vi "TOP画面.vi"() -> ()   [LabVIEW 2021]
uses:
  <vilib>/Utility/config.llb/Read Key (String).vi
  <vilib>/Utility/config.llb/NI_LVConfig.lvlib
panel:
  out "iniフォルダパス取得 2":path
  out "ini error in (no error) 2":errorcluster caption="エラー入力（エラーなし）"
  out "品番設定_品番品名1":T1
  in  "ini error in (no error)":errorcluster caption="エラー入力（エラーなし）"
  out "iniフォルダパス取得":path
  in  "品番5":bool
  in  "品番8":bool
  in  "品番7":bool
  in  "品番6":bool
  in  "品番4":bool
  in  "品番3":bool
  in  "品番2":bool
  in  "品番1":bool
  out "エラー出力":errorcluster
  in  "終了":bool
  in  "設定画面へ":bool
  # "ゲージ測定データ収集アプリ"
  # "-"
  # "品番"
  # "品名"
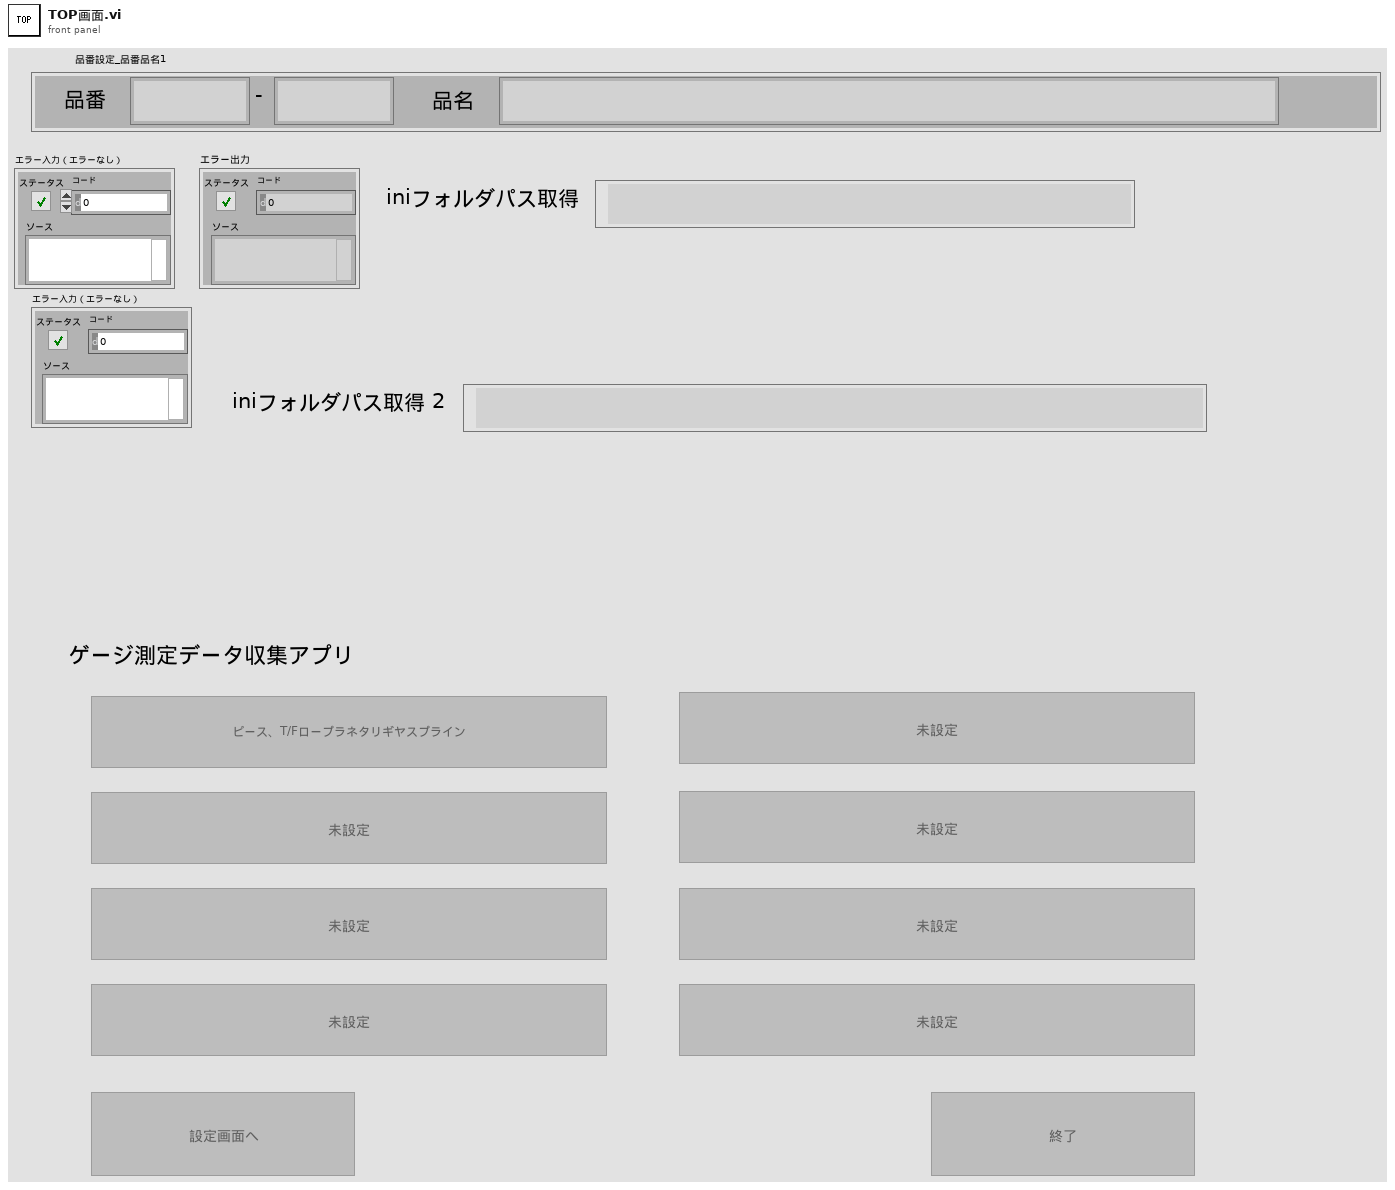
[diagram p1: front panel]
types:
  T1 = typedef "品番・品名選択用.ctl" = cluster{"品名":string, "品番前":string, "品番後":string}
  T2 = enum8{"Enabled", "Disabled", "Disabled and Grayed Out"}
  T3 = typedef "NI_LVConfig.lvlib/Config Data RefNum.ctl" = refnum<k1>
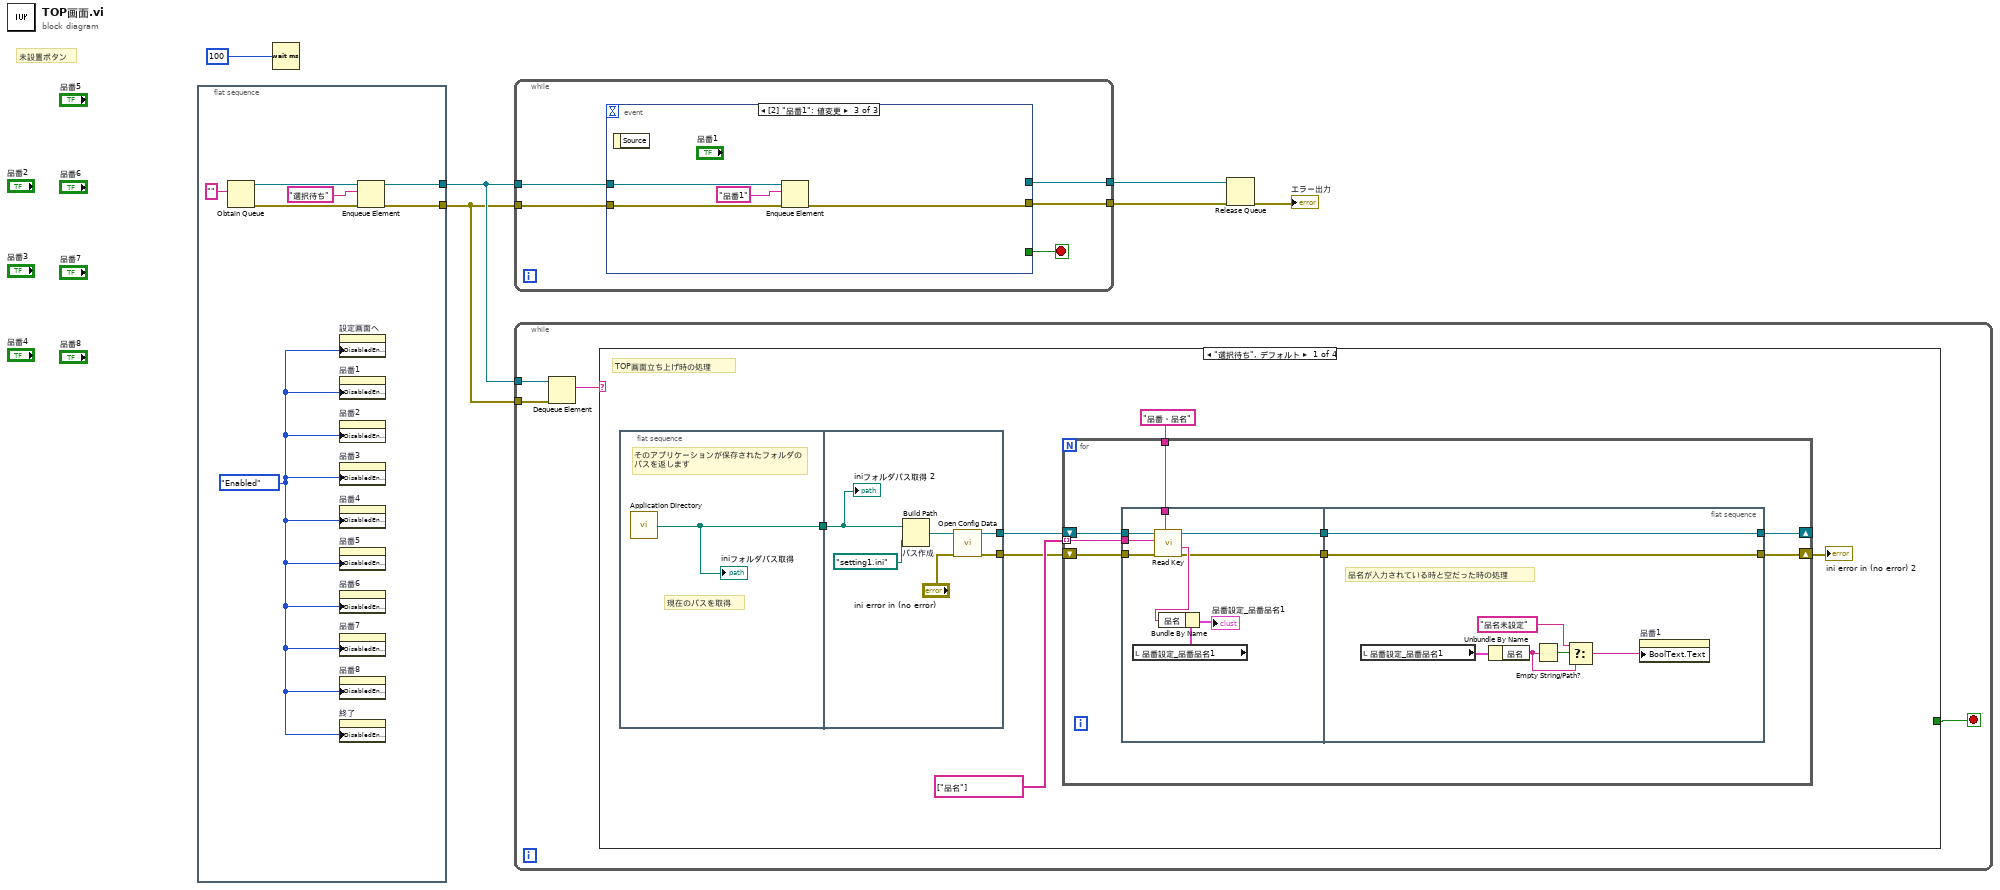
[diagram p0: block diagram]
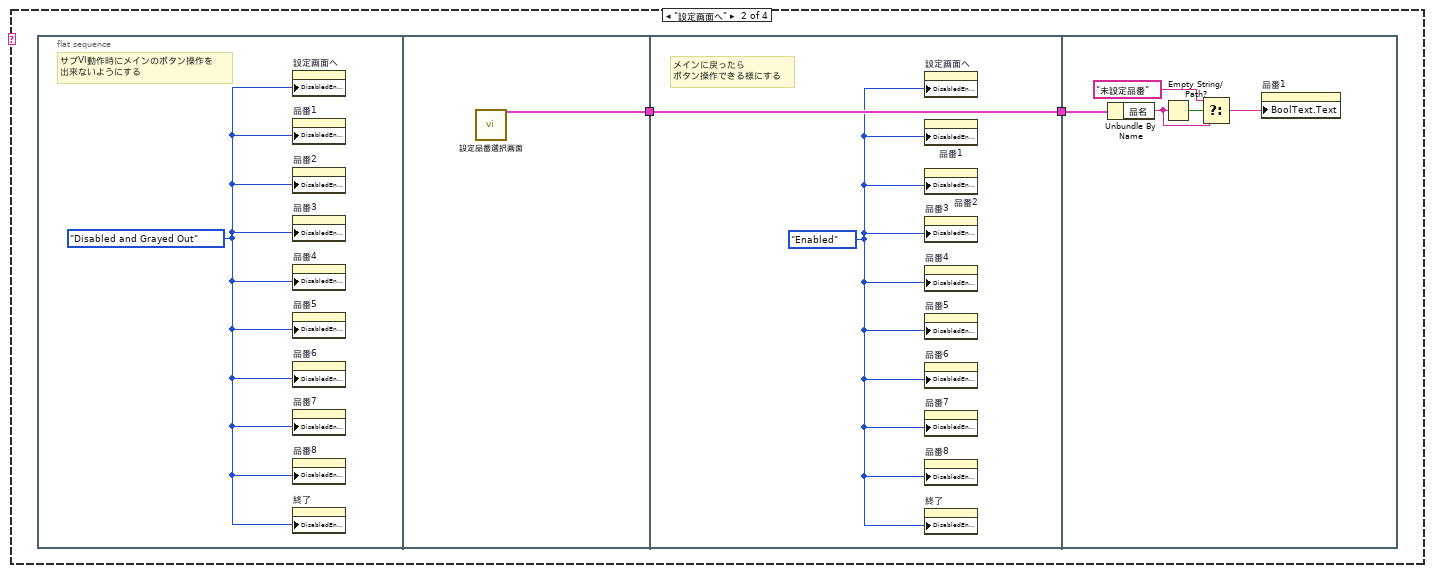
[diagram p2: hidden frame]
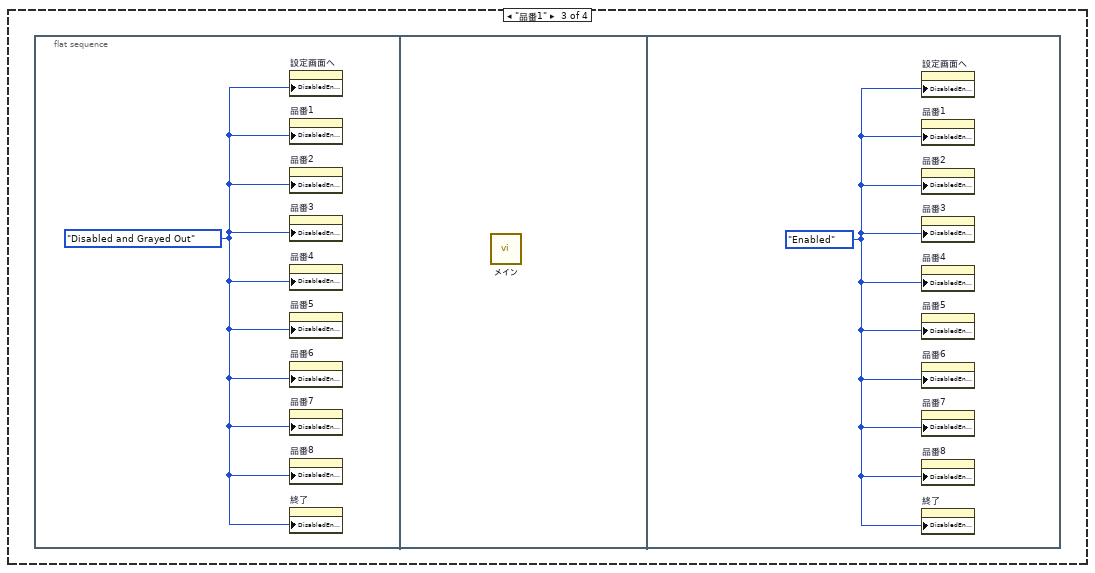
[diagram p3: hidden frame]
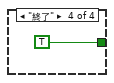
[diagram p4: hidden frame]
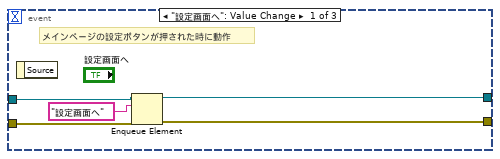
[diagram p5: hidden frame]
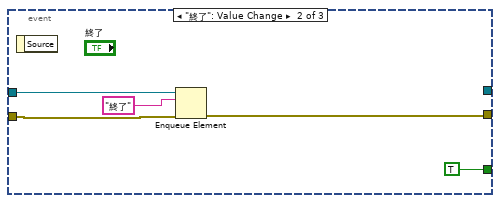
[diagram p6: hidden frame]
diagram:
  # "未設置ボタン"
  n1 = flat-sequence {
    tunnel: [w10] -> w6
    tunnel: [w8] -> w2
    frame #0 {
      w7 = T2."Enabled" ("無効")
      n2 = Obtain Queue(element data type="") -> (queue out=w12:refnum<queue>, error out=w9:errorcluster)  [unwired: 4 in, 1 out]
      n3 = property on="設定画面へ" class="Bool"("DisabledEnum"=w7) -> ()  [unwired: 2 in, 2 out]
      n4 = property on="品番1" class="Bool"("DisabledEnum"=w7) -> ()  [unwired: 2 in, 2 out]
      n5 = property on="品番2" class="Bool (指定)"("DisabledEnum"=w7) -> ()  [unwired: 2 in, 2 out]
      n6 = property on="品番3" class="Bool (指定)"("DisabledEnum"=w7) -> ()  [unwired: 2 in, 2 out]
      n7 = property on="品番4" class="Bool (指定)"("DisabledEnum"=w7) -> ()  [unwired: 2 in, 2 out]
      n8 = property on="品番5" class="Bool (指定)"("DisabledEnum"=w7) -> ()  [unwired: 2 in, 2 out]
      n9 = property on="品番6" class="Bool (指定)"("DisabledEnum"=w7) -> ()  [unwired: 2 in, 2 out]
      n10 = property on="品番7" class="Bool (指定)"("DisabledEnum"=w7) -> ()  [unwired: 2 in, 2 out]
      n11 = property on="品番8" class="Bool (指定)"("DisabledEnum"=w7) -> ()  [unwired: 2 in, 2 out]
      n12 = property on="終了" class="Bool"("DisabledEnum"=w7) -> ()  [unwired: 2 in, 2 out]
      n13 = Enqueue Element(queue=w12, element="選択待ち", error in (no error)=w9) -> (queue out=w10:refnum<queue>, error out=w8:errorcluster)  [unwired: 1 in, 1 out]
    }
  }
  n14 = Wait (ms)(milliseconds to wait=100) -> ()  [unwired: 1 out]
  n15 = while {
    tunnel: w6 -> [w18]
    tunnel: [w16] -> w5
    tunnel: w2 -> [w15]
    tunnel: [w14] -> w4
    stop <- w17 stop-if-true
    n16 = event shown="[2] \"品番1\": 値変更" {
      selector: _ -> [_ _ _]
      dyn-events: _ -> [_ _ _]
      timeout: _ -> [_ _ _]
      tunnel: w18 -> [w23 w28 w31]
      tunnel: [_ TRUE _] -> w17
      tunnel: [w21 _ _] -> w16
      tunnel: w15 -> [w20 w25 w30]
      tunnel: [w19 w24 w29] -> w14
      event "設定画面へ": Value Change {
        # "メインページの設定ボタンが押された時に動作"
        n17 = event-data() -> ()  [unwired: 1 in, 1 out]
        n18 = Enqueue Element(queue=w23, element="設定画面へ", error in (no error)=w20) -> (queue out=w21:refnum<queue>, error out=w19:errorcluster)  [unwired: 1 in, 1 out]
      }
      event "終了": Value Change {
        n19 = event-data() -> ()  [unwired: 1 in, 1 out]
        n20 = Enqueue Element(queue=w28, element="終了", error in (no error)=w25) -> (error out=w24:errorcluster)  [unwired: 1 in, 2 out]
      }
      event "品番1": Value Change {
        n21 = event-data() -> ()  [unwired: 1 in, 1 out]
        n22 = Enqueue Element(queue=w31, element="品番1", error in (no error)=w30) -> (error out=w29:errorcluster)  [unwired: 1 in, 2 out]
      }
    }
  }
  n23 = while {
    tunnel: w6 -> [w36]
    tunnel: w2 -> [w33]
    stop <- w34 stop-if-true
    n24 = Dequeue Element(queue=w36, error in (no error)=w33) -> (element=w35:string)  [unwired: 1 in, 3 out]
    n25 = case shown="\"選択待ち\", デフォルト" w35 {
      tunnel: [_ _ _ TRUE] -> w34
      frame "選択待ち", Default {
        # "TOP画面立ち上げ時の処理"
        n26 = flat-sequence {
          tunnel: [w43] -> w39
          tunnel: w39 -> [w44]
          tunnel: [w46] -> w38
          tunnel: [w45] -> w37
          frame #0 {
            # "そのアプリケーションが保存されたフォルダの\nパスを返します"
            # "現在のパスを取得"
            n27 = call <vilib>:"Application Directory.vi"() -> ("Application Directory"=w43:path)
            "iniフォルダパス取得" <- w43
          }
          frame #1 {
            n28 = Build Path "パス作成"(base path=w44, name or relative path=path "setting1.ini") -> (appended path=w49:path)
            n29 = call <vilib>:"Open Config Data.vi"("error in (no error)"="ini error in (no error)", "configuration file path"=w49) -> ("error out"=w45:errorcluster, "refnum"=w46:T3)  [unwired: 1 in, 7 out]
            "iniフォルダパス取得 2" <- w44
          }
        }
        n30 = for {
          shift-right: [w56] -> _
          shift-left: w38 -> [w57]
          tunnel: string[] ["品名"] -> [w55] mode=indexing
          tunnel: "品番・品名" -> [w54]
          shift-right: [w52] -> w41
          shift-left: w37 -> [w53]
          n31 = flat-sequence {
            tunnel: w54 -> [w63]
            tunnel: w57 -> [w62]
            tunnel: w55 -> [w61]
            tunnel: w53 -> [w60]
            tunnel: [w59] -> w51
            tunnel: [w58] -> w50
            tunnel: [w72] -> w52
            tunnel: [w73] -> w56
            tunnel: w51 -> [w73]
            tunnel: w50 -> [w72]
            frame #0 {
              n32 = local read "品番設定_品番品名1"() -> (w64:T1)
              n33 = call-poly <vilib>:"Read Key.vi"("section"=w63, "error in (no error)"=w60, "key"=w61, "refnum"=w62) -> ("error out"=w58:errorcluster, "value"=w65:string, "refnum out"=w59:T3)  [unwired: 4 in, 1 out]
              n34 = Bundle By Name(cluster=w64, "品名"=w65) -> (→"品番設定_品番品名1":T1)
            }
            frame #1 {
              # "品名が入力されている時と空だった時の処理"
              n35 = local read "品番設定_品番品名1"() -> (w71:T1)
              n36 = Unbundle By Name(w71) -> ("品名"=w69:string)
              n37 = Empty String/Path?(string/path=w69) -> (empty?=w70:bool)
              n38 = Select(t="品名未設定", s=w70, f=w69) -> (s? t:f=w67:string)
              n39 = property on="品番1" class="Bool"("BoolText.Text"=w67) -> ()  [unwired: 2 in, 2 out]
            }
          }
        }
        "ini error in (no error) 2" <- w41
      }
      frame "設定画面へ" {
        n40 = flat-sequence {
          tunnel: [w77] -> w75
          tunnel: w75 -> [w79]
          tunnel: [w79] -> w74
          tunnel: w74 -> [w84]
          frame #0 {
            w76 = T2."Disabled and Grayed Out" ("無効")
            # "サブVI動作時にメインのボタン操作を\n出来ないようにする"
            n41 = property on="設定画面へ" class="Bool"("DisabledEnum"=w76) -> ()  [unwired: 2 in, 2 out]
            n42 = property on="品番1" class="Bool"("DisabledEnum"=w76) -> ()  [unwired: 2 in, 2 out]
            n43 = property on="品番2" class="Bool (指定)"("DisabledEnum"=w76) -> ()  [unwired: 2 in, 2 out]
            n44 = property on="品番3" class="Bool (指定)"("DisabledEnum"=w76) -> ()  [unwired: 2 in, 2 out]
            n45 = property on="品番4" class="Bool (指定)"("DisabledEnum"=w76) -> ()  [unwired: 2 in, 2 out]
            n46 = property on="品番5" class="Bool (指定)"("DisabledEnum"=w76) -> ()  [unwired: 2 in, 2 out]
            n47 = property on="品番6" class="Bool (指定)"("DisabledEnum"=w76) -> ()  [unwired: 2 in, 2 out]
            n48 = property on="品番7" class="Bool (指定)"("DisabledEnum"=w76) -> ()  [unwired: 2 in, 2 out]
            n49 = property on="品番8" class="Bool (指定)"("DisabledEnum"=w76) -> ()  [unwired: 2 in, 2 out]
            n50 = property on="終了" class="Bool"("DisabledEnum"=w76) -> ()  [unwired: 2 in, 2 out]
          }
          frame #1 {
            n51 = call "設定品番選択画面.vi"() -> ("品番設定_品番品名"=w77:T1)  [unwired: 27 in]
          }
          frame #2 {
            w78 = T2."Enabled" ("無効")
            # "メインに戻ったら\nボタン操作できる様にする"
            n52 = property on="設定画面へ" class="Bool"("DisabledEnum"=w78) -> ()  [unwired: 2 in, 2 out]
            n53 = property on="品番1" class="Bool"("DisabledEnum"=w78) -> ()  [unwired: 2 in, 2 out]
            n54 = property on="品番2" class="Bool (指定)"("DisabledEnum"=w78) -> ()  [unwired: 2 in, 2 out]
            n55 = property on="品番3" class="Bool (指定)"("DisabledEnum"=w78) -> ()  [unwired: 2 in, 2 out]
            n56 = property on="品番4" class="Bool (指定)"("DisabledEnum"=w78) -> ()  [unwired: 2 in, 2 out]
            n57 = property on="品番5" class="Bool (指定)"("DisabledEnum"=w78) -> ()  [unwired: 2 in, 2 out]
            n58 = property on="品番6" class="Bool (指定)"("DisabledEnum"=w78) -> ()  [unwired: 2 in, 2 out]
            n59 = property on="品番7" class="Bool (指定)"("DisabledEnum"=w78) -> ()  [unwired: 2 in, 2 out]
            n60 = property on="品番8" class="Bool (指定)"("DisabledEnum"=w78) -> ()  [unwired: 2 in, 2 out]
            n61 = property on="終了" class="Bool"("DisabledEnum"=w78) -> ()  [unwired: 2 in, 2 out]
          }
          frame #3 {
            n62 = Unbundle By Name(w84) -> ("品名"=w81:string)
            n63 = Empty String/Path?(string/path=w81) -> (empty?=w83:bool)
            n64 = Select(t="未設定品番", s=w83, f=w81) -> (s? t:f=w80:string)
            n65 = property on="品番1" class="Bool"("BoolText.Text"=w80) -> ()  [unwired: 2 in, 2 out]
          }
        }
      }
      frame "品番1" {
        n66 = flat-sequence {
          frame #0 {
            w85 = T2."Disabled and Grayed Out" ("無効")
            n67 = property on="設定画面へ" class="Bool"("DisabledEnum"=w85) -> ()  [unwired: 2 in, 2 out]
            n68 = property on="品番1" class="Bool"("DisabledEnum"=w85) -> ()  [unwired: 2 in, 2 out]
            n69 = property on="品番2" class="Bool (指定)"("DisabledEnum"=w85) -> ()  [unwired: 2 in, 2 out]
            n70 = property on="品番3" class="Bool (指定)"("DisabledEnum"=w85) -> ()  [unwired: 2 in, 2 out]
            n71 = property on="品番4" class="Bool (指定)"("DisabledEnum"=w85) -> ()  [unwired: 2 in, 2 out]
            n72 = property on="品番5" class="Bool (指定)"("DisabledEnum"=w85) -> ()  [unwired: 2 in, 2 out]
            n73 = property on="品番6" class="Bool (指定)"("DisabledEnum"=w85) -> ()  [unwired: 2 in, 2 out]
            n74 = property on="品番7" class="Bool (指定)"("DisabledEnum"=w85) -> ()  [unwired: 2 in, 2 out]
            n75 = property on="品番8" class="Bool (指定)"("DisabledEnum"=w85) -> ()  [unwired: 2 in, 2 out]
            n76 = property on="終了" class="Bool"("DisabledEnum"=w85) -> ()  [unwired: 2 in, 2 out]
          }
          frame #1 {
            n77 = call "メイン.vi"() -> ()  [unwired: 9 in, 2 out]
          }
          frame #2 {
            w86 = T2."Enabled" ("無効")
            n78 = property on="設定画面へ" class="Bool"("DisabledEnum"=w86) -> ()  [unwired: 2 in, 2 out]
            n79 = property on="品番1" class="Bool"("DisabledEnum"=w86) -> ()  [unwired: 2 in, 2 out]
            n80 = property on="品番2" class="Bool (指定)"("DisabledEnum"=w86) -> ()  [unwired: 2 in, 2 out]
            n81 = property on="品番3" class="Bool (指定)"("DisabledEnum"=w86) -> ()  [unwired: 2 in, 2 out]
            n82 = property on="品番4" class="Bool (指定)"("DisabledEnum"=w86) -> ()  [unwired: 2 in, 2 out]
            n83 = property on="品番5" class="Bool (指定)"("DisabledEnum"=w86) -> ()  [unwired: 2 in, 2 out]
            n84 = property on="品番6" class="Bool (指定)"("DisabledEnum"=w86) -> ()  [unwired: 2 in, 2 out]
            n85 = property on="品番7" class="Bool (指定)"("DisabledEnum"=w86) -> ()  [unwired: 2 in, 2 out]
            n86 = property on="品番8" class="Bool (指定)"("DisabledEnum"=w86) -> ()  [unwired: 2 in, 2 out]
            n87 = property on="終了" class="Bool"("DisabledEnum"=w86) -> ()  [unwired: 2 in, 2 out]
          }
        }
      }
      frame "終了" {
      }
    }
  }
  n88 = Release Queue(queue=w5, error in (no error)=w4) -> (error out=→"エラー出力":errorcluster)  [unwired: 1 in, 2 out]
